vi "autoDrive.vi"(0 "Distance to Travel":dbl=-4.0) -> (2 "finished?":bool, 3 "left speed":dbl, 4 "right speed":dbl)   [LabVIEW 2013]
doc: "Will drive the robot at a specified speed for a specified distance. Pretty simple."
uses:
  typedefs/State Machine/subStates.ctl
  typedefs/fg_typedef.ctl
  <vilib>/addons/control/pid/pid.llb/PID (DBL).vi
  <vilib>/addons/control/pid/NI_PID_pid.lvlib
panel:
  out "leftRate":dbl
  out "rightRate":dbl
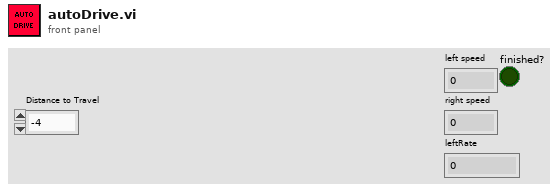
[diagram p1: front panel]
types:
  T1 = cluster{"proportional gain (Kc)":dbl, "integral time (Ti, min)":dbl, "derivative time (Td, min)":dbl}
  T2 = typedef "fg_typedef.ctl" = enum16{"Get", "Set"}
  T3 = typedef "subStates.ctl" = enum16{"null", "wait", "driver control", "auto", "manual override", "hold position", "rotate", "pickup", "pass", "load", "goto shoot", "shoot high goal", "shoot low goal", "cancel arm", "cancel shooter", "end", "test"}
  T4 = typedef "WPI_EncoderDevRef.ctl" = cluster{"DevStatus":errorcluster, "EncoderIndex":T5, "CounterIndex":T6, "DistancePerCount":dbl, "Decoding Type":T7}
  T5 = typedef "FPGA_EncoderIdx.ctl" = enum8{"Enc 0", "Enc 1", "Enc 2", "Enc 3", "Invalid"}
  T6 = typedef "FPGA_CounterCtrSystemIndex.ctl" = enum8{"Ctr 0", "Ctr 1", "Ctr 2", "Ctr 3", "Ctr 4", "Ctr 5", "Ctr 6", "Ctr 7", "Invalid"}
  T7 = typedef "WPI_EncoderType.ctl" = enum16{"1x", "2x", "4x"}
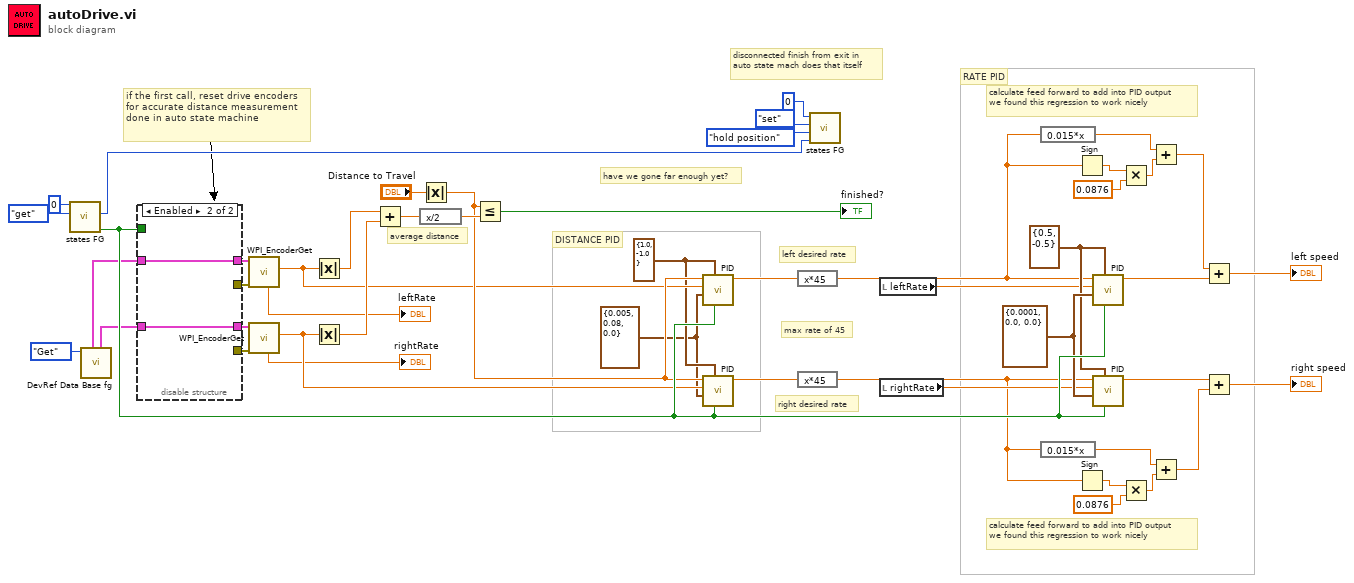
[diagram p0: block diagram]
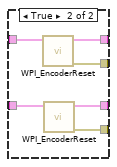
[diagram p3: hidden frame]
diagram:
  w21 = cluster{"output high":dbl, "output low":dbl} {"output high"=1.0, "output low"=-1.0} ("output range")
  w20 = T1 {"proportional gain (Kc)"=0.005, "integral time (Ti, min)"=0.08, "derivative time (Td, min)"=0.0} ("PID gains")
  w25 = T1 {"proportional gain (Kc)"=0.0001, "integral time (Ti, min)"=0.0, "derivative time (Td, min)"=0.0} ("PID gains")
  w15 = cluster{"output high":dbl, "output low":dbl} {"output high"=0.5, "output low"=-0.5} ("output range")
  # "RATE PID"
  # "DISTANCE PID"
  # "disconnected finish from exit in\nauto state mach does that itself"
  # "calculate feed forward to add into PID output\nwe found this regression to work nicely"
  # "calculate feed forward to add into PID output\nwe found this regression to work nicely"
  # "max rate of 45"
  # "left desired rate"
  # "right desired rate"
  # "if the first call, reset drive encoders for accurate distance measurement\ndone in auto state machine"
  # "have we gone far enough yet?"
  # "average distance"
  n1 = call "states FG.vi"("menu (get)"=enum16{"set", "get"}."get", "Loop ID"=0) -> ("first call?"=w49:bool, "state # out"=w33:i32)  [unwired: 6 in, 2 out]
  n2 = call "DevRef Data Base fg.vi"("Menu"=fg_typedef."Get") -> ("right drive encoder"=w27:T4, "left drive encoder"=w28:T4)  [unwired: 3 in, 4 out]
  n3 = disable-structure shown="Enabled" {
    disable-tunnel: w28 -> [w56 w66]
    disable-tunnel: w27 -> [w55 w65]
    disable-tunnel: [w54 _] -> w41
    disable-tunnel: [w53 w66] -> w40
    disable-tunnel: [w52 w65] -> w39
    disable-tunnel: [w51 _] -> w38
    disable-tunnel: w49 -> [w50 _]
    frame Disabled {
      n4 = case shown="False" w50 {
        tunnel: w56 -> [w58 w63]
        tunnel: w55 -> [w57 w61]
        tunnel: [_ w64] -> w54
        tunnel: [w58 w62] -> w53
        tunnel: [w57 w60] -> w52
        tunnel: [_ w59] -> w51
        frame False {
        }
        frame True {
          n5 = call <vilib>:"WPI_EncoderReset.vi"("EncoderDevRef"=w63) -> ("error out"=w64:errorcluster, "EncoderDevRef"=w62:T4)  [unwired: 9 in]
          n6 = call <vilib>:"WPI_EncoderReset.vi"("EncoderDevRef"=w61) -> ("error out"=w59:errorcluster, "EncoderDevRef"=w60:T4)  [unwired: 9 in]
        }
      }
    }
    frame Enabled {
    }
  }
  n7 = call <vilib>:"WPI_EncoderGet.vi"("error in (no error)"=w41, "EncoderDevRef"=w40) -> ("Distance"=w31:dbl, "Rate"=→"leftRate":dbl)  [unwired: 4 in, 4 out]
  n8 = call <vilib>:"WPI_EncoderGet.vi"("error in (no error)"=w38, "EncoderDevRef"=w39) -> ("Distance"=w30:dbl, "Rate"=→"rightRate":dbl)  [unwired: 4 in, 4 out]
  n9 = Absolute Value(x=w31) -> (abs(x)=w35:dbl)
  n10 = Absolute Value(x=w30) -> (abs(x)=w34:dbl)
  n11 = Add(x=w35, y=w34) -> (x+y=w47:dbl)
  n12 = expression code="x/2"(w47) -> (w46:dbl)
  n13 = Absolute Value(x="Distance to Travel") -> (abs(x)=w32:dbl)
  n14 = Less Or Equal?(x=w32, y=w46) -> (x <= y?=→"finished?":bool)
  n15 = call-poly <vilib>:"PID.vi"("reinitialize? (F)"=w49, "output range"=w21, "PID gains"=w20, "process variable"=w31, "setpoint"=w32) -> ("output"=w23:dbl)  [unwired: 5 in, 1 out]
  n16 = call-poly <vilib>:"PID.vi"("reinitialize? (F)"=w49, "output range"=w21, "PID gains"=w20, "process variable"=w30, "setpoint"=w32) -> ("output"=w22:dbl)  [unwired: 5 in, 1 out]
  n17 = expression code="x*45"(w23) -> (w5:dbl)
  n18 = expression code="x*45"(w22) -> (w12:dbl)
  n19 = call "states FG.vi"("state # in"=w33, "subState in"=subStates."hold position", "menu (get)"=enum16{"set", "get"}."set", "Loop ID"=0) -> ()  [unwired: 4 in, 4 out]
  n20 = local read "leftRate"() -> (w14:dbl)
  n21 = local read "rightRate"() -> (w13:dbl)
  n22 = expression code="0.015*x"(w5) -> (w8:dbl)
  n23 = expression code="0.015*x"(w12) -> (w4:dbl)
  n24 = Sign(1:w5) -> (0:w11:dbl)
  n25 = Sign(1:w12) -> (0:w1:dbl)
  n26 = call-poly <vilib>:"PID.vi"("reinitialize? (F)"=w49, "output range"=w15, "PID gains"=w25, "process variable"=w14, "setpoint"=w5) -> ("output"=w7:dbl)  [unwired: 5 in, 1 out]
  n27 = call-poly <vilib>:"PID.vi"("reinitialize? (F)"=w49, "output range"=w15, "PID gains"=w25, "process variable"=w13, "setpoint"=w12) -> ("output"=w24:dbl)  [unwired: 5 in, 1 out]
  n28 = Multiply(x=w11, y=0.0876) -> (x*y=w9:dbl)
  n29 = Multiply(x=w1, y=0.0876) -> (x*y=w3:dbl)
  n30 = Add(x=w8, y=w9) -> (x+y=w6:dbl)
  n31 = Add(x=w4, y=w3) -> (x+y=w26:dbl)
  n32 = Add(x=w6, y=w7) -> (x+y=→"left speed":dbl)
  n33 = Add(x=w24, y=w26) -> (x+y=→"right speed":dbl)
